vi "PH_Beamline.PC _PABypass.vi"(0 "i ref in":refnum<vi>, 2 "Service Name":string="N/A", 3 "Value":i32, 4 "no link?":bool, 5 "error in (no error)":errorcluster) -> (14 "i ref out":refnum<vi>, 19 "error out":errorcluster)   [LabVIEW 2009, in "PH_Beamline.lvlib"]
doc: "This VI writes the incoming information for Laser-, PreAmp- and MainAmp-Freigabe to the related GUI element and to own attributes."
uses:
  PH_Beamline.lvlib
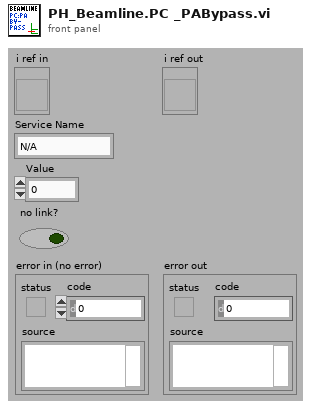
[diagram p1: front panel]
types:
  T1 = typedef "PH_Beamline.lvlib/PH_Beamline.i attribute.ctl" = cluster{"GUI Refs":cluster{"Delete":refnum<vi>, "BL ok":refnum<vi>, "PA ok":refnum<vi>, "MA ok":refnum<vi>, "fs FE ok":refnum<vi>, "ns FE ok":refnum<vi>, "PA ED ok":refnum<vi>, "MAS ok":refnum<vi>, "Booster ok":refnum<vi>, "Mirrortower ok":refnum<vi>, "In.-Box ok":refnum<vi>, "Compressor ok":refnum<vi>, "Experiment LB ok":refnum<vi>, "Experiment LL ok":refnum<vi>, "PHELIX_Beckhoff_Watchdog":refnum<vi>, "Shutters closed":refnum<vi>}, "Beamline State":cluster{"Subsystems":cluster{"PA":bool, "MA":bool, "ns FE":bool, "fs FE":bool, "PA ED":bool, "In.-Box":bool, "MAS":bool, "Booster":bool, "Mirrortower":bool, "Compressor":bool, "Experiment LB":bool, "Experiment LL":bool}, "State":bool}, "Remote Controlled by":string, "R2S ID":i32, "Refs BL MA":refnum<vi>[], "Refs Motion":refnum<vi>[], "Refs Cams":refnum<vi>[], "Refs Ops":refnum<vi>[], "State BBs":T2[], "Refs BBs":refnum<vi>[], "State Switches":T2[], "Refs Switches":refnum<vi>[], "Refs Vac":refnum<vi>[], "Vacua":cluster{"Instance":string, "Channelname":string, "Limit":dbl, "Curr Value":dbl, "in range":bool}[], "Refs BL MA-IB":refnum<vi>[], "Refs BL fs":refnum<vi>[], "Refs BL PA ED":refnum<vi>[], "Refs BL MAS":refnum<vi>[], "Refs Powermeter":refnum<vi>[], "Refs O2":refnum<vi>[], "O2 Inspection":cluster{"Concentration":dbl, "State":T2}[], "Refs BL Boo":refnum<vi>[], "Refs BL ns":refnum<vi>[], "Refs BL Mirrortower":refnum<vi>[], "Refs BL Compressor":refnum<vi>[], "Refs BL Exp LB":refnum<vi>[], "Refs 6P Switches":refnum<vi>[], "State 6P Switches":T2[], "Radiation Safety":cluster{"Exp Laserbay":cluster{"Ref Op Mode":refnum<vi>, "Ref Laserbay evacuated":refnum<vi>, "Tagname LB evacuated":string, "Shot Mode":T3, "Laserbay evacuated?":i32, "Tagname HV room locked":string, "HV room locked?":i32, "Ref HV room locked":refnum<vi>, "Tagname bridged?":string, "Ref Bridge":refnum<vi>, "I<1E18W/cm²":bool}, "Exp Laserlab":cluster{"Ref Op Mode":refnum<vi>, "Ref Laserlab evacuated":refnum<vi>, "Tagname LL evacuated":string, "Shot Mode":T3, "Laserlab evacuated?":i32, "Tagname bridged?":string, "Ref Bridge":refnum<vi>, "I<1E18W/cm²":bool}}, "Refs Switch and Motion":refnum<vi>[], "State Switch and Motion":T2[], "GUI manager Path":string, "Refs BL LL":refnum<vi>[], "Refs Switch GUI":refnum<vi>[], "State Switch GUIs":bool[], "Refs Spectrometer":refnum<vi>[], "PP Igni Heating GUI Refs":refnum<vi>[], "PP Igni Heating Tagnames ":string[], "Refs local GUIs":refnum<vi>[], "Refs BL PA":cluster{"undelayed Line before Shutter":refnum<vi>[], "undelayed Line after Shutter":refnum<vi>[], "before Bypass":refnum<vi>[], "delayed Line before Shutter":refnum<vi>[], "delayed Line after Shutter":refnum<vi>[], "before Shutter Input":refnum<vi>[], "after Shutter Input":refnum<vi>[], "Bypass":refnum<vi>[], "before Shutter Exit":refnum<vi>[], "after Shutter Exit":refnum<vi>[], "to MA":refnum<vi>[], "to Lab":refnum<vi>[]}, "Refs SSACs":refnum<vi>[], "Service ID":cluster{"YLF_BL_Status":i32, "fs_BL_Status":i32, "fs_YLF_BL_Status":i32, "ns_BL_Status":i32, "PA_Input_BL_Status":i32, "PA_UnDelay_BL_Status":i32, "PA_Delay_BL_Status":i32, "PA_BL_Status":i32, "PA_Bypass_BL_Status":i32, "PA_Exit_BL_Status":i32, "PA_LL_BL_Status":i32, "LL_BL_Status":i32, "PA_MA_BL_Status":i32, "MA_Exit_BL_Status":i32, "MA_Z6_BL_Status":i32, "Z6_BL_Status":i32, "MA_LB_BL_Status":i32, "LB_TB2_BL_Status":i32, "PA_before_Bypass_BL_Status":i32, "LB_TB3_BL_Status":i32}, "BL":cluster{"YLF_BL_Status":i32, "fs_BL_Status":i32, "fs_YLF_BL_Status":i32, "ns_BL_Status":i32, "PA_Input_BL_Status":i32, "PA_UnDelay_BL_Status":i32, "PA_Delay_BL_Status":i32, "PA_BL_Status":i32, "PA_Bypass_BL_Status":i32, "PA_Exit_BL_Status":i32, "PA_LL_BL_Status":i32, "LL_BL_Status":i32, "PA_MA_BL_Status":i32, "MA_Exit_BL_Status":i32, "MA_Z6_BL_Status":i32, "Z6_BL_Status":i32, "MA_LB_BL_Status":i32, "LB_TB2_BL_Status":i32, "PA_before_Bypass_BL_Status":i32, "LB_TB3_BL_Status":i32}, "Refs Existance Booleans":refnum<vi>[], "Refs free Motion GUIs":refnum<vi>[], "Refs Crosshairs":refnum<vi>[]}
  T2 = typedef "Status.ctl" = i16
  T3 = typedef "Operation Mode.ctl" = i32
  T4 = enum16{"No Link", "No Info", "In", "Out", "in between"}
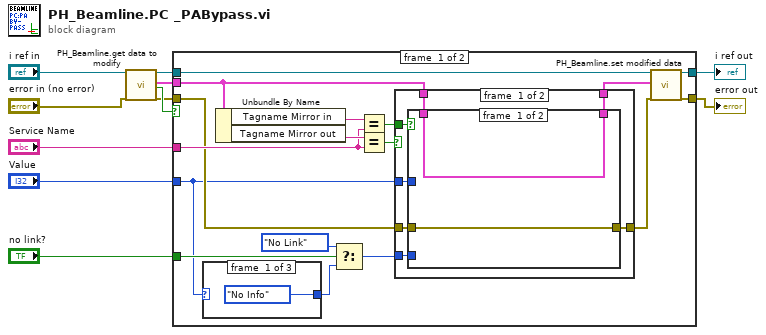
[diagram p0: block diagram]
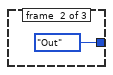
[diagram p2: hidden frame]
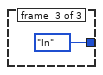
[diagram p3: hidden frame]
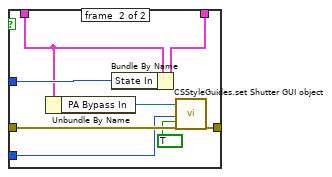
[diagram p4: hidden frame]
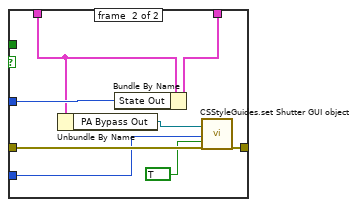
[diagram p5: hidden frame]
diagram:
  n1 = call "PH_Beamline.get data to modify.vi"("i ref in"="i ref in", "error in (no error)"="error in (no error)") -> ("i ref out"=w6:refnum<vi>, "i attribute"=w10:T1, "timed out"=w11:bool, "error out"=w8:errorcluster)  [unwired: 14 in]
  n2 = case shown="False" w11 {
    tunnel: w6 -> [w28 w58]
    tunnel: [w27 w58] -> w7
    tunnel: w8 -> [w19 w57]
    tunnel: [w20 w57] -> w9
    tunnel: w10 -> [w21 _]
    tunnel: "Value" -> [w14 _]
    tunnel: "Service Name" -> [w22 _]
    tunnel: "no link?" -> [w17 _]
    frame #0 {
      n3 = case shown="0, Default" w14 {
        tunnel: [T4."No Info" ("Shutter State") T4."Out" ("Shutter State") T4."In" ("Shutter State")] -> w13
        frame #0 {
        }
        frame #1 {
        }
        frame #2 {
        }
      }
      n4 = Unbundle By Name(w21) -> ("Tagname Mirror in"=w25:string, "Tagname Mirror out"=w26:string)
      n5 = Select(t=T4."No Link" ("Shutter State"), s=w17, f=w13) -> (s? t:f=w15:T4)
      n6 = Equal?(x=w25, y=w22) -> (x = y?=w23:bool)
      n7 = Equal?(x=w26, y=w22) -> (x = y?=w24:bool)
      n8 = case shown="False" w24 {
        tunnel: w23 -> [w38 _]
        tunnel: w21 -> [w37 w54]
        tunnel: [w36 w56] -> w12
        tunnel: w14 -> [w35 w55]
        tunnel: w19 -> [w34 w52]
        tunnel: [w33 w51] -> w18
        tunnel: w15 -> [w32 w50]
        frame #0 {
          n9 = case shown="True" w38 {
            tunnel: w37 -> [w40 w44]
            tunnel: [w40 w48] -> w36
            tunnel: w35 -> [_ w47]
            tunnel: w34 -> [w39 w46]
            tunnel: [w39 w45] -> w33
            tunnel: w32 -> [_ w42]
            frame #0 {
            }
            frame #1 {
              n10 = Unbundle By Name(w44) -> ("PA Bypass In"=w43:refnum<vi>)
              n11 = Bundle By Name(cluster=w44, "State In"=w47) -> (w48:T1)
              n12 = call "CSStyleGuides.set Shutter GUI object.vi"("Ref Object"=w43, "Shutter State"=w42, "Disabled? (false)"=TRUE, "error in (no error)"=w46) -> ("error out"=w45:errorcluster)  [unwired: 15 in]
            }
          }
        }
        frame #1 {
          n13 = Unbundle By Name(w54) -> ("PA Bypass Out"=w53:refnum<vi>)
          n14 = Bundle By Name(cluster=w54, "State Out"=w55) -> (w56:T1)
          n15 = call "CSStyleGuides.set Shutter GUI object.vi"("Ref Object"=w53, "Shutter State"=w50, "Disabled? (false)"=TRUE, "error in (no error)"=w52) -> ("error out"=w51:errorcluster)  [unwired: 15 in]
        }
      }
      n16 = call "PH_Beamline.set modified data.vi"("i ref in"=w28, "i attribute"=w12, "error in (no error)"=w18) -> ("i ref out"=w27:refnum<vi>, "error out"=w20:errorcluster)  [unwired: 15 in]
    }
    frame #1 {
    }
  }
  "error out" <- w9
  "i ref out" <- w7
